vi "Add Device.vi"(8 "error in (no error)":errorcluster, 10 "Device":refnum<class "Device.lvclass">, 11 "HAL Editor in":refnum<class "HAL Editor.lvclass">) -> (0 "error out":errorcluster, 3 "HAL Editor out":refnum<class "HAL Editor.lvclass">)   [LabVIEW 2012, in "HAL Config.lvlib" / "HAL Editor.lvclass"]
uses:
  HAL Editor.lvclass
  build/ppl/lv-hal.lvlibp/Device/Device.lvclass
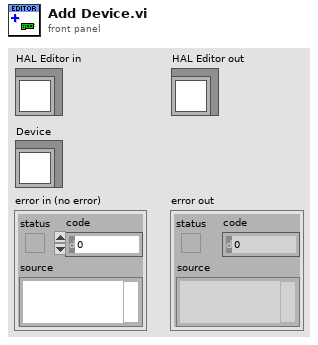
[diagram p1: front panel]
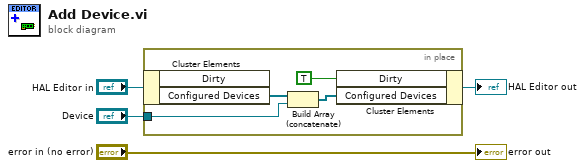
[diagram p0: block diagram]
diagram:
  n1 = in-place {
    in-place-border: "Device" -> [w7]
    n2 = in-place-cluster #1("HAL Editor in") -> ("Configured Devices"=w8:refnum<class "Device.lvclass">[])  [unwired: 1 out]
    n3 = Build Array (concatenate)(w8, w7) -> (w6:refnum<class "Device.lvclass">[])
    n4 = in-place-cluster #1("Dirty"=TRUE, "Configured Devices"=w6) -> (→"HAL Editor out":refnum<class "HAL Editor.lvclass">)
  }
  "error out" <- "error in (no error)"
